vi "put_pdo_node.vi"(10 "node":u8, 11 "index":u16) -> (3 "return":i16)   [LabVIEW 2011]
uses:
  canopen_dll_master.dll
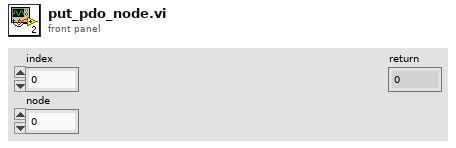
[diagram p1: front panel]
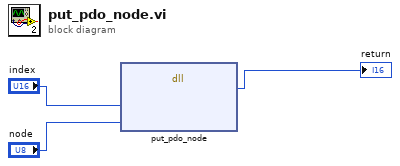
[diagram p0: block diagram]
diagram:
  n1 = dll-call lib="canopen_dll_master.dll" fn="put_pdo_node"("index"="index", "node"="node") -> ("return type"=→"return":i16)  [unwired: 5 in, 2 out]
